vi "multimeter reader.vi"() -> ()   [LabVIEW 2012, in "multimeter reader.lvclass"]
uses:
  multimeter reader.lvclass
  Reader/Reader.lvclass
panel:
  in  "Reader.lvclass":refnum<class "Reader.lvclass">
  in  "multimeter reader.lvclass":refnum<class "multimeter reader.lvclass">
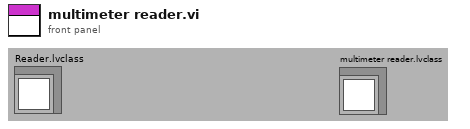
[diagram p1: front panel]
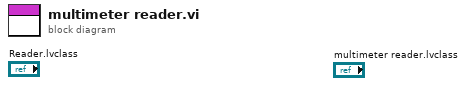
[diagram p0: block diagram]
diagram:
